vi "Cal Dir.vi"(0 "Lifter_motor in":refnum<class "Lifter_motor.lvclass">, 1 "Step In range":bool, 5 "Possition selector":T1(radio), 7 "Step Distance":dbl, 9 "ADC distance":dbl, 11 "error in (no error)":errorcluster) -> (4 "Lifter_motor out":refnum<class "Lifter_motor.lvclass">, 6 "Direction":bool, 15 "error out":errorcluster)   [LabVIEW 2019, in "Lifter_motor.lvclass"]
uses:
  Lifter_motor.lvclass
  Lifter_motor.lvclass/Lifter_motor.ctl
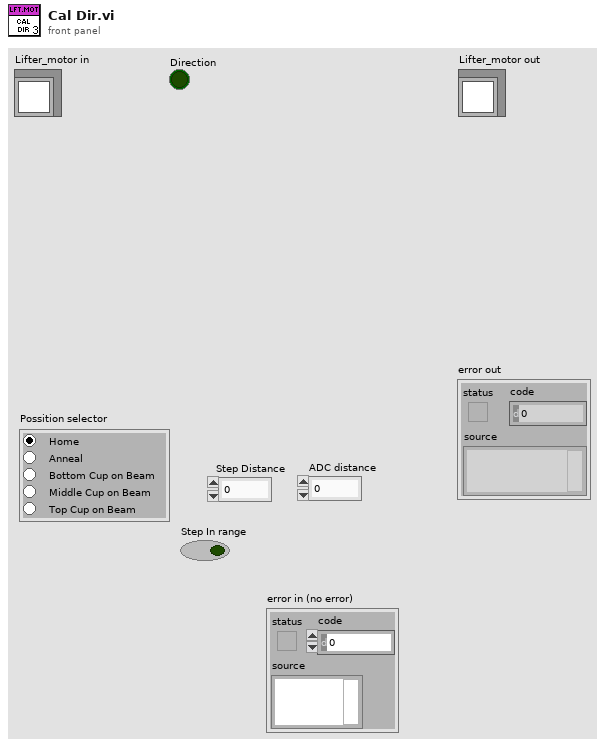
[diagram p1: front panel]
types:
  T1 = enum32{"Home", "Anneal", "Bottom Cup on Beam", "Middle Cup on Beam", "Top Cup on Beam"}
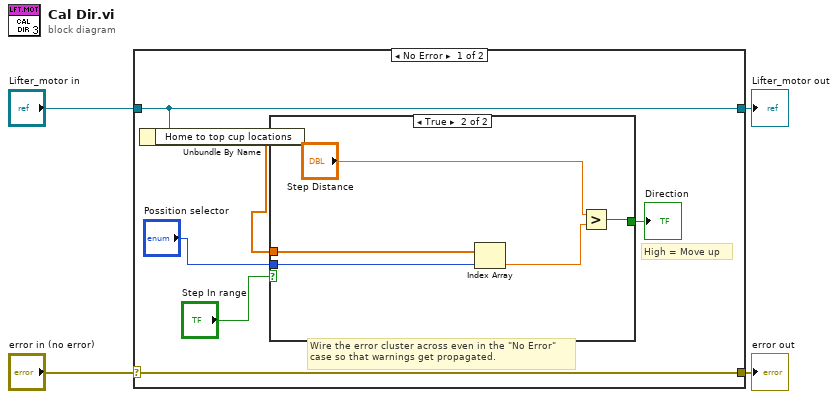
[diagram p0: block diagram]
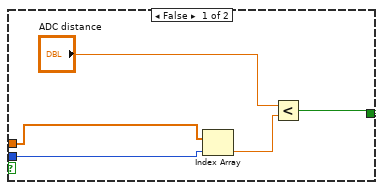
[diagram p2: hidden frame]
diagram:
  n1 = case shown="No Error" "error in (no error)" {
    selector: "error in (no error)" -> [w10 w22]
    tunnel: [w10 w22] -> w3
    tunnel: [w6 w21] -> w1
    tunnel: "Lifter_motor in" -> [w6 w21]
    frame No Error {
      # "High = Move up"
      # "Wire the error cluster across even in the \"No Error\"\ncase so that warnings get propagated."
      n2 = Unbundle By Name(w6) -> ("Home to top cup locations"=w5:dbl[])
      n3 = case shown="True" "Step In range" {
        tunnel: [w14 w20] -> w7
        tunnel: "Possition selector" -> [w12 w18]
        tunnel: w5 -> [w11 w16]
        frame False {
          n4 = Index Array(array=w11, index=w12) -> (element=w13:dbl)
          n5 = Less?(x="ADC distance", y=w13) -> (x < y?=w14:bool)
        }
        frame True {
          n6 = Index Array(array=w16, index=w18) -> (element=w17:dbl)
          n7 = Greater?(x="Step Distance", y=w17) -> (0:w20:bool)
        }
      }
      "Direction" <- w7
    }
    frame Error {
    }
  }
  "error out" <- w3
  "Lifter_motor out" <- w1
